vi "Write RP I-V Configuration.vi"(8 "error in (no error)":errorcluster, 10 "Configuration":T1={"I-V parameters"={"Start magnitude"=2e-05, "Magnitude increment"=5e-05, "End magnitude"=50.0, "Ramp length"=0, "Top  length"=0, "Threshold "=2e-06, "Processing delay"=255, "Valhalla range"=0.001, "Interpolation"=64, "Stop after"=1, "Detector window"=480}, "Ranges"=[1.0, 1.0], "Pre-trigger duration"=0.01, "Post-trigger duration"=0.1, "Output delay"=0.1} {"Output delay" format="%#_6ps"; "Post-trigger duration" format="%#_6ps"; "Pre-trigger duration" format="%#_6ps"; "Ranges" format="%#_6pV"; "I-V parameters"."Detector window" format="%dpts"; "I-V parameters"."Stop after" format="%d sweep(s)"; "I-V parameters"."Valhalla range" format="%#_6pA"; "I-V parameters"."Processing delay" format="%dpts"; "I-V parameters"."Threshold" format="%#_6pV"; "I-V parameters"."Top  length" format="%dpts"; "I-V parameters"."Ramp length" format="%dpts"; "I-V parameters"."End magnitude" format="%#_6pA"; "I-V parameters"."Magnitude increment" format="%#_6pA"; "I-V parameters"."Start magnitude" format="%#_6pA"}, 11 "RP I-V in":refnum<class "RP I-V.lvclass">) -> (0 "error out":errorcluster, 3 "RP I-V out":refnum<class "RP I-V.lvclass">)   [LabVIEW 2018, in "RP I-V.lvclass"]
uses:
  RP I-V.lvclass
  C:/github/LabActor/Template Module/Template Module.lvclass
  NHMFL_Core/Libraries/Red Pitaya/RP Core/Rep Pitaya I-V driver/RP I-V Configuration.ctl
  NHMFL_Core/Libraries/Red Pitaya/Waform generation/I-V parameters.ctl
  Template Module/Template Module.lvclass/Template Module.ctl
  Template Module/Write Configuration.vi
panel:
  # "Waveform parameters"
  # "Detector parameters"
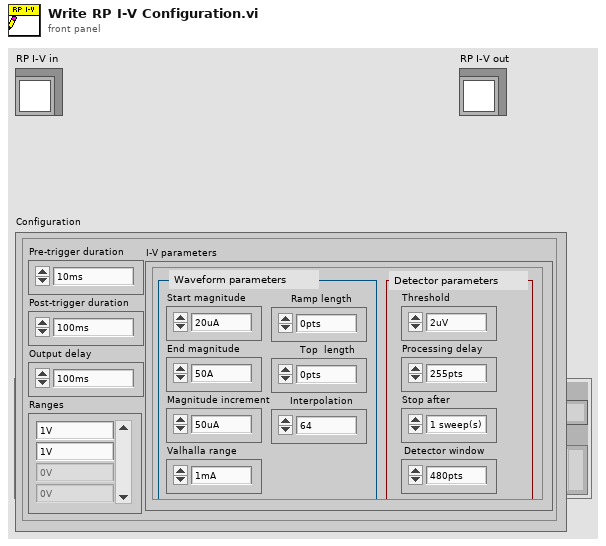
[diagram p1: front panel]
types:
  T1 = typedef "RP I-V Configuration.ctl" = cluster{"I-V parameters":T2, "Ranges":dbl[], "Pre-trigger duration":dbl, "Post-trigger duration":dbl, "Output delay":dbl}
  T2 = typedef "I-V parameters.ctl" = cluster{"Start magnitude":dbl, "Magnitude increment":dbl, "End magnitude":dbl, "Ramp length":i32, "Top  length":i32, "Threshold ":dbl, "Processing delay":u16, "Valhalla range":dbl, "Interpolation":i32, "Stop after":u16, "Detector window":i32}
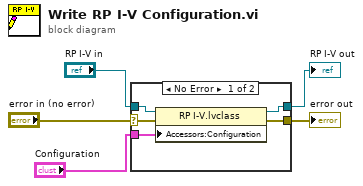
[diagram p0: block diagram]
diagram:
  n1 = case shown="No Error" "error in (no error)" {
    selector: "error in (no error)" -> [w7 w11]
    tunnel: [w6 w11] -> w1
    tunnel: [w8 w12] -> w5
    tunnel: "RP I-V in" -> [w9 w12]
    tunnel: "Configuration" -> [w10 _]
    frame No Error {
      n2 = property class="RP I-V.lvclass"(reference=w9, error in=w7, "Accessors:Configuration"=w10) -> (reference out=w8:refnum<class "RP I-V.lvclass">, error out=w6:errorcluster)
    }
    frame Error {
    }
  }
  "error out" <- w1
  "RP I-V out" <- w5
